vi "Last Ack.vi"(10 "Actor":refnum<class "Actor.lvclass">, 11 "jettl Queue Actor in":refnum<class "jettl Queue Actor.lvclass">) -> (3 "jettl Queue Actor out":refnum<class "jettl Queue Actor.lvclass">)   [LabVIEW 2021, in "jettl Queue Actor.lvlib" / "jettl Queue Actor.lvclass"]
uses:
  jettl Queue Actor.lvclass
  Actor/Actor/Actor.lvclass
  C:/git/jettl/src/Actor/Actor/Actor.lvclass
  C:/git/jettl/src/Actor/Msgs/Setup/Setup/Setup.lvclass
  C:/git/jettl/src/Actor/Msgs/Teardown/Teardown/Teardown.lvclass
  C:/git/jettl/src/Actor/Queue Actor/Queue Actor.lvclass
  C:/git/jettl/src/Actor/Msgs/Event Create/Event Create/Event Create.lvclass
  C:/git/jettl/src/Actor/Msgs/Event Last Ack/Event Last Ack/Event Last Ack.lvclass
  C:/git/jettl/src/Actor/Msgs/Queue Create/Queue Create/Queue Create.lvclass
  C:/git/jettl/src/Actor/Msgs/Queue Last Ack/Queue Last Ack/Queue Last Ack.lvclass
  C:/git/jettl/src/jettl/jettl Queue Actor/jettl Queue Actor/jettl Queue Actor.lvclass
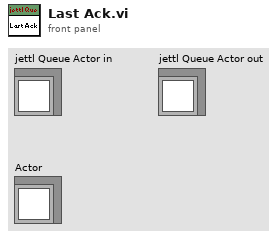
[diagram p1: front panel]
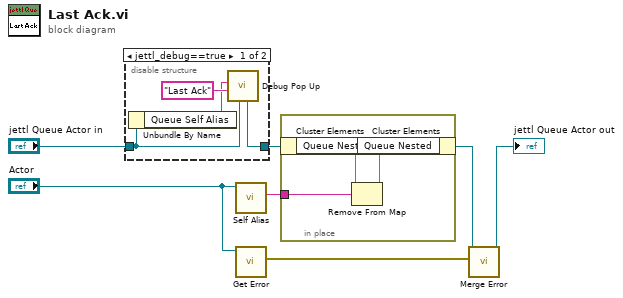
[diagram p0: block diagram]
diagram:
  n1 = disable-structure shown="jettl_debug==true" {
    disable-tunnel: "jettl Queue Actor in" -> [w9 _]
    disable-tunnel: [w10 _] -> w3
    frame condition #0 (active) {
      n2 = Unbundle By Name(w9) -> ("Queue Self Alias"=w8:string)
      n3 = call "Debug Pop Up.vi"("Input"=w9, "Method"="Last Ack", "Alias"=w8) -> ("Output"=w10:refnum<class "jettl Queue Actor.lvclass">)  [unwired: 8 in]
    }
    frame condition #1 {
    }
  }
  n4 = call-dynamic "Self Alias.vi"("Actor in"="Actor") -> ("Self Alias"=w6:string)  [unwired: 10 in]
  n5 = call-dynamic "Get Error.vi"("Actor in"="Actor") -> ("Error"=w5:errorcluster)  [unwired: 10 in]
  n6 = in-place {
    in-place-border: w6 -> [w12]
    n7 = in-place-cluster #1(w3) -> ("Queue Nested"=w13:map{string, refnum<data-value>})
    n8 = Remove From Map(10:w12, 11:w13) -> (3:w14:map{string, refnum<data-value>})  [unwired: 2 out]
    n9 = in-place-cluster #1("Queue Nested"=w14) -> (w4:refnum<class "jettl Queue Actor.lvclass">)
  }
  n10 = call-dynamic "Merge Error.vi"("Error"=w5, "jettl Queue Actor in"=w4) -> ("jettl Queue Actor out"=→"jettl Queue Actor out":refnum<class "jettl Queue Actor.lvclass">)  [unwired: 9 in]
